vi "ge_EditINT.vi"(4 "CellSize":T3, 6 "ActiveCellPos":T1, 7 "String Value":string, 8 "error in":errorcluster, 11 "FP Ctrl":T2) -> (0 "error out":errorcluster, 1 "Discard?":bool)   [LabVIEW 2018]
uses:
  <vilib>/Utility/miscctls.llb/LVBoundsTypeDef.ctl
  Custom Ctrls/ge_FPCtrlRefLabel.ctl
  <vilib>/Utility/miscctls.llb/LVPositionTypeDef.ctl
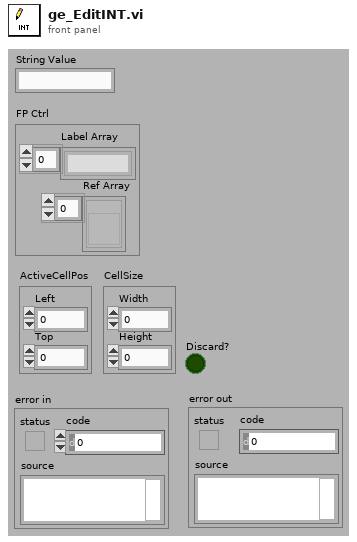
[diagram p1: front panel]
types:
  T1 = typedef "LVPositionTypeDef.ctl" = cluster{"Left":i32, "Top":i32}
  T2 = typedef "ge_FPCtrlRefLabel.ctl" = cluster{"Label Array":string[], "Ref Array":refnum<vi>[]}
  T3 = typedef "LVBoundsTypeDef.ctl" = cluster{"Width":u32, "Height":u32}
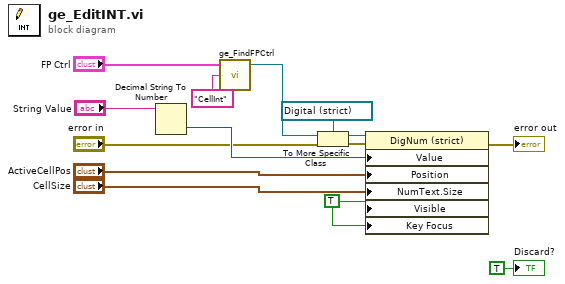
[diagram p0: block diagram]
diagram:
  w9 = TRUE ("Visible")
  n1 = Decimal String To Number(string="String Value") -> (number=w10:i32)  [unwired: 2 in, 1 out]
  n2 = call "ge_FindFPCtrl.vi"("Ctrl Name"="CellInt" ("Name"), "FP Ctrl"="FP Ctrl") -> ("Ctrl Ref"=w7:refnum<vi>)  [unwired: 3 in]
  n3 = To More Specific Class(target class=refnum<vi> refnum ("reference"), reference=w7, error in="error in") -> (specific class reference=w4:refnum<vi>, error out=w5:errorcluster)
  n4 = property on="Property Node" class="DigNum (strict)"(reference=w4, error in=w5, "Value"=w10, "Position"="ActiveCellPos", "NumText.Size"="CellSize", "Visible"=w9, "Key Focus"=w9) -> (error out=→"error out":errorcluster)  [unwired: 1 out]
  "Discard?" <- TRUE ("Discard?")
